vi "daqtest.vi"() -> ()   [LabVIEW 2015]
uses:
  <vilib>/Waveform/WDTOps.llb/WDT Append Waveforms DBL.vi
  <vilib>/Waveform/WDTOps.llb/WDT Waveform Duration DBL.vi
  <vilib>/Waveform/WDTFileIO.llb/Export Waveform To Spreadsheet File.vi
panel:
  in  "stop":bool
  out "Waveform Chart":waveform(dbl)(graph)
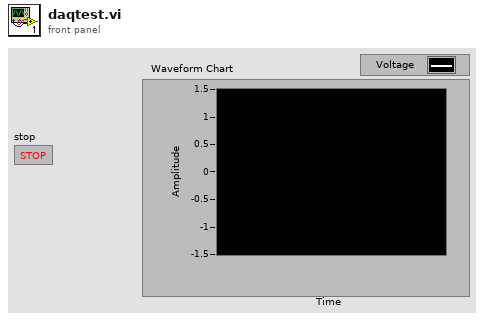
[diagram p1: front panel]
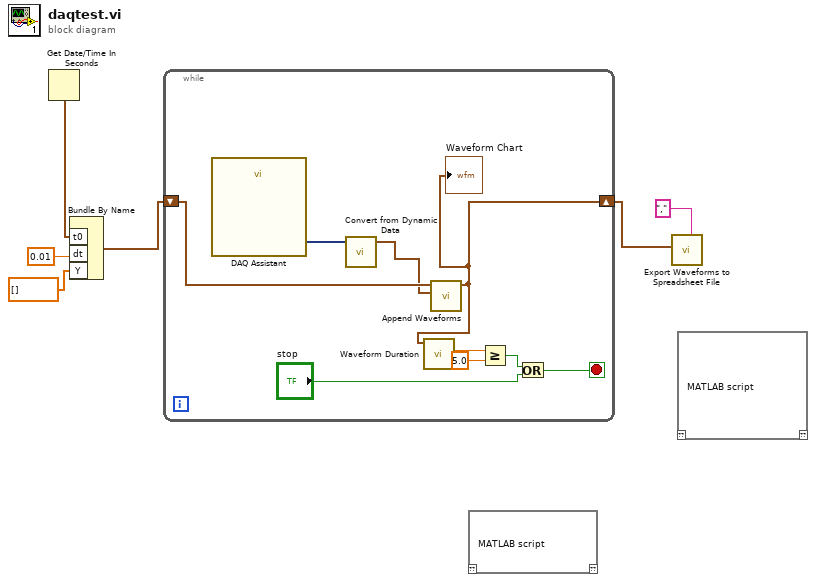
[diagram p0: block diagram]
diagram:
  n1 = Get Date/Time In Seconds() -> (seconds since 1Jan1904=w4:timestamp)
  n2 = Bundle By Name("t0"=w4, "dt"=0.01, "Y"=dbl[] []) -> (w3:waveform(dbl))  [unwired: 1 in]
  n3 = while {
    shift-right: [w12] -> w2
    shift-left: w3 -> [w14]
    stop <- w7 stop-if-true
    n4 = call "DAQ Assistant"() -> ("data"=w15:dynamicdata)  [unwired: 17 in, 2 out]
    n5 = call "Convert from Dynamic Data"("Dynamic Data Type"=w15) -> ("Waveform"=w13:waveform(dbl))  [unwired: 3 in]
    n6 = call-poly <vilib>:"Append Waveforms.vi"("waveform B"=w13, "waveform A"=w14) -> ("waveform out"=w12:waveform(dbl))  [unwired: 8 in, 1 out]
    "Waveform Chart" <- w12
    n7 = call-poly <vilib>:"Waveform Duration.vi"("waveform in"=w12) -> ("duration"=w11:dbl)  [unwired: 8 in, 2 out]
    n8 = Greater Or Equal?(x=w11, y=5.0) -> (x >= y?=w9:bool)
    n9 = Or(x=w9, y="stop") -> (x .or. y?=w7:bool)
  }
  n10 = script code="MATLAB script"() -> ()  [unwired: 1 in, 1 out]
  n11 = call-poly <vilib>:"Export Waveforms to Spreadsheet File.vi"("delimiter (Tab)"=",", "waveform"=w2) -> ()  [unwired: 8 in, 2 out]
  n12 = script code="MATLAB script"() -> ()  [unwired: 1 in, 1 out]
